vi "Get google_protobuf_Option.vi"(8 "error in (no error)":errorcluster, 11 "gRPCid":T3) -> (0 "error out":errorcluster, 2 "package_templatemessage":T1, 3 "gRPCid out":T3)   [LabVIEW 2020, in "LineRegulation.lvlib"]
uses:
  LineRegulation.lvlib
  <vilib>/gRPC/LabVIEW gRPC Library/Shared/grpcId.ctl
  google_protobuf_Option.ctl
  google_protobuf_Any.ctl
  a51dd2a7-b5c1-4c09-9df4-8cd9d3bd0c19.vi
  <vilib>/gRPC/LabVIEW gRPC Library/Shared/TranslateGrpcError.vi
  <vilib>/gRPC/LabVIEW gRPC Library/Server API/Server/Get Server DLL Path.vi
  <vilib>/Utility/error.llb/Error Cluster From Error Code.vi
  <vilib>/gRPC/LabVIEW gRPC Library/grpc-lvsupport-release.lvlib
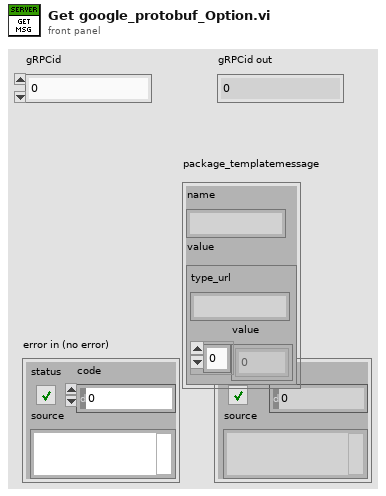
[diagram p1: front panel]
types:
  T1 = typedef "LineRegulation.lvlib/google_protobuf_Option.ctl" = cluster{"name":string, "value":T2}
  T2 = typedef "LineRegulation.lvlib/google_protobuf_Any.ctl" = cluster{"type_url":string, "value":u8[]}
  T3 = typedef "grpc-lvsupport-release.lvlib/grpcId.ctl" = u64
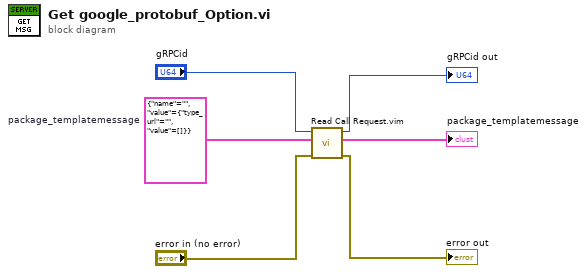
[diagram p0: block diagram]
diagram:
  w2 = T1 {"name"="", "value"={"type_url"="", "value"=[]}}  # package_templatemessage
  n1 = call "Read Call Request.vim"("error in"="error in (no error)", "Request Type"=w2, "gRPCid in"="gRPCid") -> ("error out"=→"error out":errorcluster, "Request Data"=→"package_templatemessage":T1, "gRPCid out"=→"gRPCid out":T3)  [unwired: 6 in]
